vi "Config_Execute_Write_TRF.vi"(0 "VISA Refnum in":refnum<visa-resource-name>, 1 "TRF Cluster in":T3, 2 "Gate Current Cluster":T7, 3 "Loop Count":dbl, 4 "Compliance Cluster":T2, 5 "Error In":errorcluster, 6 "Saved Folder:":path, 7 "Graph Cluster":T6, 8 "Sample Properties:":T8, 9 "Dielectric Constant (BG)":dbl, 10 "SMU4? (Y/N)":bool, 11 "Ambient Temp (Y/N)":bool, 13 "SMU Config":T1={"Vname"="Vs", "Vname 2"="Vd", "Vname 3"="Vg", "Vname 4"="V4", "Iname"="Is", "Iname 2"="Id", "Iname 3"="Ig", "Iname 4"="I4", "Mode"=4, "Mode 2"=0, "Mode 3"=0, "Mode 4"=0, "Function"=4, "Function 2"=2, "Function 3"=1, "Function 4"=4, "Value (V or A)"=0.0, "Value (Either V or A) 2"=0.0, "Value (Either V or A) 3"=0.0, "Value (Either V or A) 4"=0.0} {"Function" items=["disabled", "Var1", "Var2", "Var1'", "Constant"]; "Mode" items=["V", "I", "VPulse", "IPulse", "Common"]; "Function 4" items=["disabled", "Var1", "Var2", "Var1'", "Constant"]; "Mode 4" items=["V", "I", "VPulse", "IPulse", "Common"]; "Function 3" items=["disabled", "Var1", "Var2", "Var1'", "Constant"]; "Mode 3" items=["V", "I", "VPulse", "IPulse", "Common"]; "Function 2" items=["disabled", "Var1", "Var2", "Var1'", "Constant"]; "Mode 2" items=["V", "I", "VPulse", "IPulse", "Common"]}) -> (12 "Filepath Out 2":path, 14 "Filepath Out":path, 15 "Check Cluster":T5, 16 "Output":T4, 17 "Graph Cluster out":T6, 18 "TRF Cluster out":T3, 19 "error out":errorcluster)   [LabVIEW 2012]
panel:
  # "SMU1"
  # "SMU2"
  # "SMU3"
  # "SMU4"
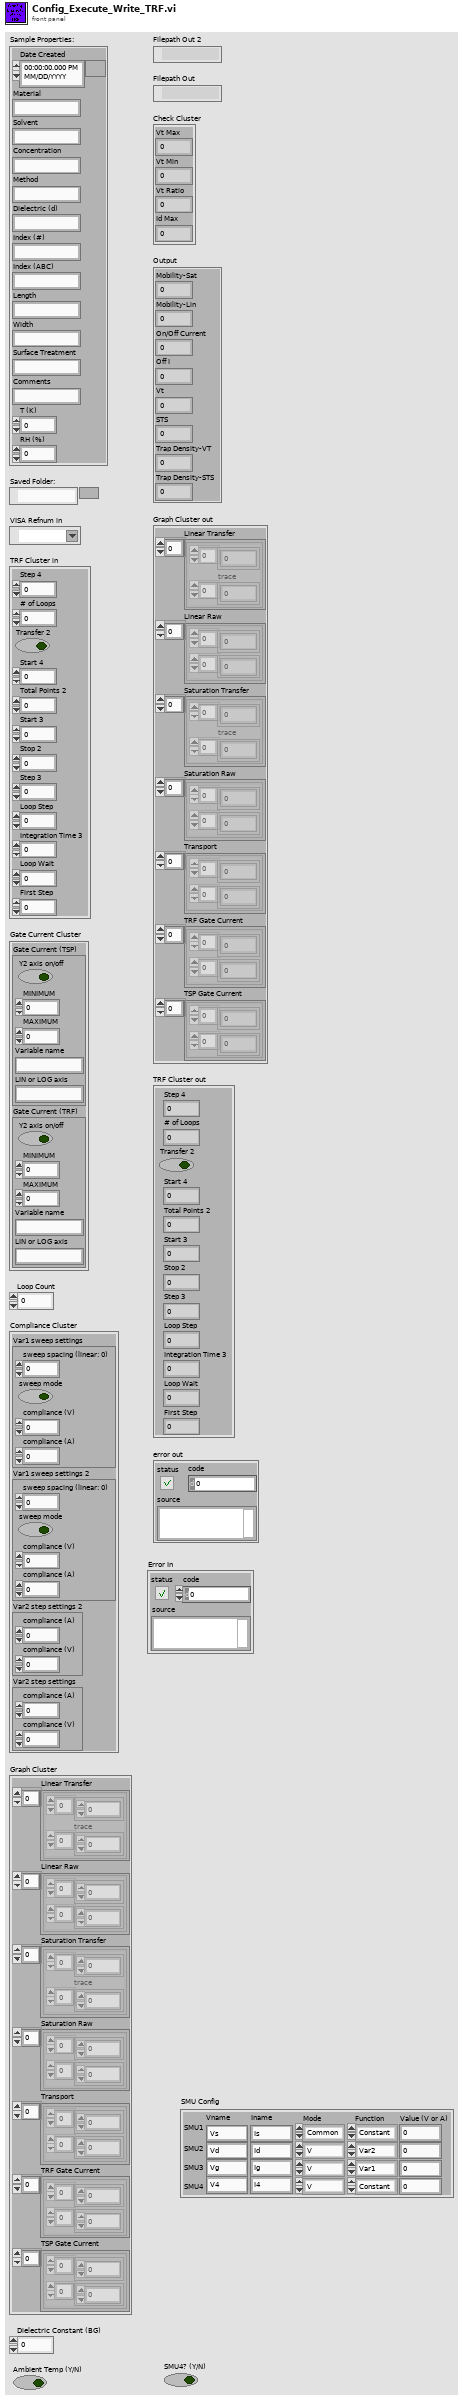
[diagram p1: front panel]
types:
  T1 = cluster{"Vname":string, "Vname 2":string, "Vname 3":string, "Vname 4":string, "Iname":string, "Iname 2":string, "Iname 3":string, "Iname 4":string, "Mode":u16, "Mode 2":u16, "Mode 3":u16, "Mode 4":u16, "Function":u16, "Function 2":u16, "Function 3":u16, "Function 4":u16, "Value (V or A)":dbl, "Value (Either V or A) 2":dbl, "Value (Either V or A) 3":dbl, "Value (Either V or A) 4":dbl}
  T2 = cluster{"Var1 sweep settings":cluster{"sweep spacing (linear: 0)":u16, "sweep mode":bool, "compliance (V)":dbl, "compliance (A)":dbl}, "Var1 sweep settings 2":cluster{"sweep spacing (linear: 0)":u16, "sweep mode":bool, "compliance (V)":dbl, "compliance (A)":dbl}, "Var2 step settings 2":cluster{"compliance (A)":dbl, "compliance (V)":dbl}, "Var2 step settings":cluster{"compliance (A)":dbl, "compliance (V)":dbl}}
  T3 = cluster{"Step 4":dbl, "# of Loops":dbl, "Transfer 2":bool, "Start 4":dbl, "Total Points 2":u16, "Start 3":dbl, "Stop 2":dbl, "Step 3":dbl, "Loop Step":dbl, "Integration Time 3":u32, "Loop Wait":dbl, "First Step":dbl}
  T4 = cluster{"Mobility-Sat":dbl, "Mobility-Lin":dbl, "On/Off Current":dbl, "Off I":dbl, "Vt":dbl, "STS":dbl, "Trap Density-VT":dbl, "Trap Density-STS":dbl}
  T5 = cluster{"Vt Max":i32, "Vt Min":i32, "Vt Ratio":i32, "Id Max":dbl}
  T6 = cluster{"Linear Transfer":cluster{dbl[], "trace":dbl[]}[], "Linear Raw":cluster{dbl[], dbl[]}[], "Saturation Transfer":cluster{dbl[], "trace":dbl[]}[], "Saturation Raw":cluster{dbl[], dbl[]}[], "Transport":cluster{dbl[], dbl[]}[], "TRF Gate Current":cluster{dbl[], dbl[]}[], "TSP Gate Current":cluster{dbl[], dbl[]}[]}
  T7 = cluster{"Gate Current (TSP)":cluster{"Y2 axis on/off":bool, "MINIMUM":ext, "MAXIMUM":ext, "Variable name":string, "LIN or LOG axis":string}, "Gate Current (TRF)":cluster{"Y2 axis on/off":bool, "MINIMUM":ext, "MAXIMUM":ext, "Variable name":string, "LIN or LOG axis":string}}
  T8 = cluster{"Date Created":timestamp, "Material":string, "Solvent":string, "Concentration":string, "Method":string, "Dielectric (d)":string, "Index (#)":string, "Index (ABC)":string, "Length":string, "Width":string, "Surface Treatment":string, "Comments":string, "T (K)":dbl, "RH (%)":dbl}
  T9 = cluster{"sweep spacing (linear: 0)":u16, "sweep mode":bool, "compliance (V)":dbl, "compliance (A)":dbl}
  T10 = cluster{"compliance (A)":dbl, "compliance (V)":dbl}
  T11 = cluster{"Start 3":dbl, "Stop 2":dbl, "Step 3":dbl, "sweep spacing (linear: 0)":u16, "sweep mode":bool, "compliance (V)":dbl, "compliance (A)":dbl}
  T12 = cluster{"Y2 axis on/off":bool, "MINIMUM":ext, "MAXIMUM":ext, "Variable name":string, "LIN or LOG axis":string}
  T13 = cluster{"compliance (A)":dbl, "compliance (V)":dbl, "Start 4":dbl, "Total Points 2":u16, dbl}
  T14 = cluster{"Linear Sqrt":cluster{dbl[], "trace":dbl[]}[], "Linear Log":cluster{dbl[], "trace":dbl[]}[], "Linear Raw":cluster{dbl[], dbl[]}[], "Saturation Sqrt":cluster{dbl[], "trace":dbl[]}[], "Saturation Log":cluster{dbl[], "trace":dbl[]}[], "Saturation Raw":cluster{dbl[], "trace":dbl[]}[], "Gate Current":cluster{dbl[], "trace":dbl[]}[]}
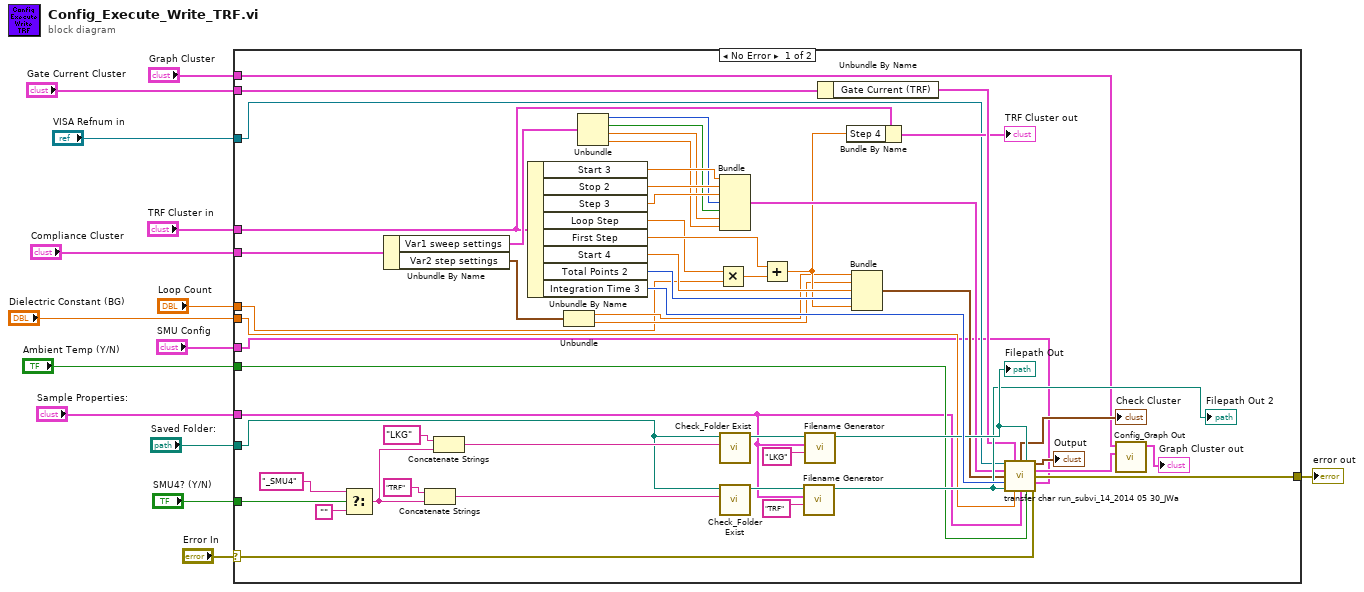
[diagram p0: block diagram]
diagram:
  n1 = case shown="No Error" "Error In" {
    selector: "Error In" -> [w27 w68]
    tunnel: [w35 w68] -> w13
    tunnel: "SMU4? (Y/N)" -> [w26 _]
    tunnel: "Loop Count" -> [w25 _]
    tunnel: "Dielectric Constant (BG)" -> [w24 _]
    tunnel: "Ambient Temp (Y/N)" -> [w23 _]
    tunnel: "Compliance Cluster" -> [w22 _]
    tunnel: "TRF Cluster in" -> [w21 _]
    tunnel: "Sample Properties:" -> [w20 _]
    tunnel: "Saved Folder:" -> [w19 _]
    tunnel: "Gate Current Cluster" -> [w18 _]
    tunnel: "VISA Refnum in" -> [w17 _]
    tunnel: "Graph Cluster" -> [w16 _]
    tunnel: "SMU Config" -> [w15 _]
    frame No Error {
      n2 = Select(t="_SMU4", s=w26, f="") -> (s? t:f=w30:string)
      n3 = Unbundle By Name(w22) -> ("Var1 sweep settings"=w46:T9, "Var2 step settings"=w45:T10)
      n4 = Concatenate Strings("TRF", w30) -> (w29:string)
      n5 = Concatenate Strings("LKG", w30) -> (w33:string)
      n6 = Unbundle By Name(w21) -> ("Start 3"=w42:dbl, "Stop 2"=w43:dbl, "Step 3"=w44:dbl, "Loop Step"=w63:dbl, "First Step"=w64:dbl, "Start 4"=w65:dbl, "Total Points 2"=w66:u16, "Integration Time 3"=w67:u32)
      n7 = Unbundle(w45) -> ("compliance (A)"=w40:dbl, "compliance (V)"=w41:dbl)
      n8 = Unbundle(w46) -> ("sweep spacing (linear: 0)"=w36:u16, "sweep mode"=w37:bool, "compliance (V)"=w38:dbl, "compliance (A)"=w39:dbl)
      n9 = Multiply(x=w63, y=w25) -> (x*y=w47:dbl)
      n10 = Bundle("Start 3"=w42, "Stop 2"=w43, "Step 3"=w44, "sweep spacing (linear: 0)"=w36, "sweep mode"=w37, "compliance (V)"=w38, "compliance (A)"=w39) -> (w50:T11)  [unwired: 1 in]
      n11 = call "Check_Folder Exist.vi"("Folder Name"=w33, "Root Folder"=w19) -> ("Output Path"=w58:path)  [unwired: 9 in]
      n12 = call "Check_Folder Exist.vi"("Folder Name"=w29, "Root Folder"=w19) -> ("Output Path"=w62:path)  [unwired: 9 in]
      n13 = Add(x=w64, y=w47) -> (x+y=w49:dbl)
      n14 = call "Filename Generator.vi"("Measurement Type"="TRF", "Sample Properties:"=w20, "Saved Folder:"=w62) -> ("Filepath Out"=w60:path)  [unwired: 8 in]
      "Filepath Out 2" <- w60
      n15 = call "Filename Generator.vi"("Measurement Type"="LKG", "Sample Properties:"=w20, "Saved Folder:"=w58) -> ("Filepath Out"=w61:path)  [unwired: 8 in]
      "Filepath Out" <- w61
      n16 = Unbundle By Name(w18) -> ("Gate Current (TRF)"=w56:T12)
      n17 = Bundle By Name(cluster=w21, "Step 4"=w49) -> (→"TRF Cluster out":T3)
      n18 = Bundle("compliance (A)"=w40, "compliance (V)"=w41, "Start 4"=w65, "Total Points 2"=w66, w49) -> (w51:T13)  [unwired: 1 in]
      n19 = call "transfer char run_subvi_14_2014 05 30_JWa.vi"("VISA session"=w17, "Y2 axis settings"=w56, "LKG Path"=w61, "Var1 sweep settings"=w50, "Var2 step settings"=w51, "integration time"=w67, "SMU Config"=w15, "Input Path"=w60, "Dielectric Constant"=w24, "Sample Properties:"=w20, "Ambient Temp (Y/N)"=w23, "Error In"=w27) -> ("Check Cluster"=→"Check Cluster":T5, "Output"=→"Output":T4, "Graph Cluster"=w54:T14, "Error Out"=w35:errorcluster)
      n20 = call "Config_Graph Out.vi"("Graph Cluster 3"=w54, "Graph Cluster in"=w16) -> ("Graph Cluster out"=→"Graph Cluster out":T6)  [unwired: 9 in]
    }
    frame Error {
    }
  }
  "error out" <- w13
